vi "ble.vi"() -> ()   [LabVIEW 2021]
uses:
  <vilib>/numeric/Random Number (Range) U64.vi
  <vilib>/numeric/sub_Random U32.vi
panel:
  out "?":dbl[](array[numeric])
  out "Waveform Graph":dbl[](graph)
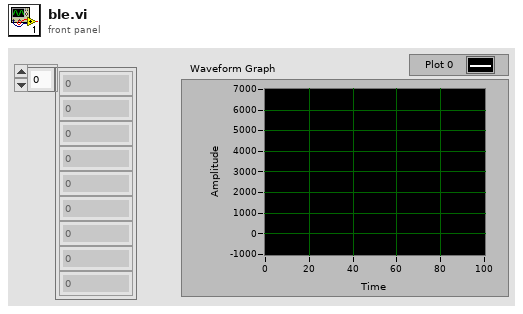
[diagram p1: front panel]
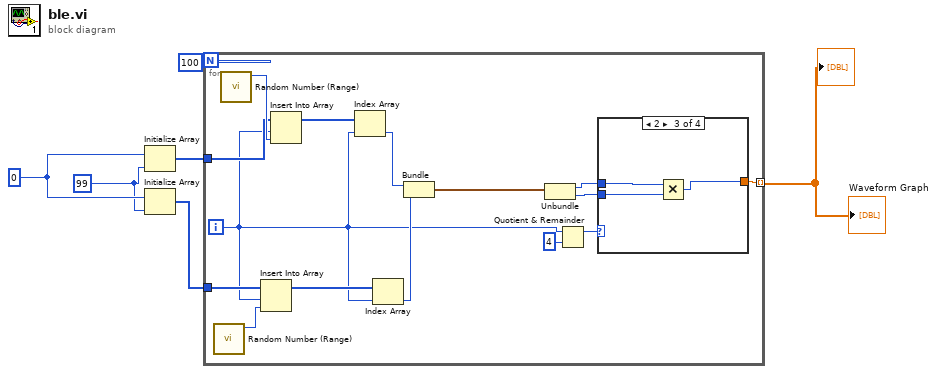
[diagram p0: block diagram]
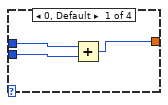
[diagram p2: hidden frame]
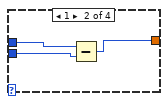
[diagram p3: hidden frame]
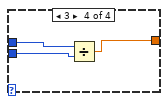
[diagram p4: hidden frame]
diagram:
  w2 = 0
  w1 = 99
  n1 = Initialize Array(w2, w1) -> (w4:i32[])
  n2 = Initialize Array(w2, w1) -> (w3:i32[])
  n3 = for {
    N: 100 -> [_]
    tunnel: [w21] -> w5 mode=indexing
    tunnel: w4 -> [w19]
    tunnel: w3 -> [w17]
    i -> [w7]
    n4 = call-poly <vilib>:"Random Number (Range).vi"() -> ("number"=w18:u64)  [unwired: 11 in]
    n5 = call-poly <vilib>:"Random Number (Range).vi"() -> ("number"=w20:u64)  [unwired: 11 in]
    n6 = Insert Into Array(array=w17, index=w7, new element=w18) -> (w16:i32[])
    n7 = Insert Into Array(array=w19, index=w7, new element=w20) -> (w15:i32[])
    n8 = Index Array(array=w15, index=w7) -> (element=w14:i32)
    n9 = Index Array(array=w16, index=w7) -> (element=w13:i32)
    n10 = Bundle(w14, w13) -> (w11:cluster{i32, i32})  [unwired: 1 in]
    n11 = Unbundle(w11) -> (w10:i32, w9:i32)
    n12 = Quotient & Remainder(x=w7, y=4) -> (x-y*floor(x/y)=w8:i32)  [unwired: 1 out]
    n13 = case shown="2" w8 {
      tunnel: w10 -> [w24 w27 w30 w33]
      tunnel: w9 -> [w23 w26 w29 w32]
      tunnel: [w22 w25 w28 w31] -> w21
      frame 0, Default {
        n14 = Add(x=w24, y=w23) -> (x+y=w22:i32)
      }
      frame 1 {
        n15 = Subtract(x=w27, y=w26) -> (x-y=w25:i32)
      }
      frame 2 {
        n16 = Multiply(x=w30, y=w29) -> (x*y=w28:i32)
      }
      frame 3 {
        n17 = Divide(x=w33, y=w32) -> (x/y=w31:dbl)
      }
    }
  }
  "Waveform Graph" <- w5
  "?" <- w5
